vi "GEA2 Write ERD.vi"(0 "GEA2 Reference In":refnum<k24>, 1 "Retry Count":i32=5, 2 "Read Timeout (ms)":u32=500, 5 "GEA Inputs":T1 {"Destination" format="%.0x"; "Source" format="%.0x"}, 7 "Write ERD List":T2[](array[typedef]) {"ERD Number" format="%.0x"}, 11 "Error In":errorcluster, 13 "Verify ERD Response?":bool=TRUE) -> (4 "GEA2 Reference Out":refnum<k24>, 6 "Raw Data Out":string, 15 "Error Out":errorcluster)   [LabVIEW 2016, in "GEA2_Toolkit.lvlib"]
doc: "This VI writes an array of ERDs with a single command. The data type is used to convert the Data from the type specified to a hexidecimal string before sending it."
uses:
  library/GEA2_Toolkit.lvlib
  type defs/ERD Write Data In.ctl
  type defs/Data Type.ctl
  type defs/Source_Destination.ctl
  C:/TechnologyLab/NI-2010/Trunk/Utility/LabVIEW GEA2 Toolkit v1.0.0.0/Appliance.NET/GeaCommunication.dll
  Appliance.NET/GeaCommunication.dll
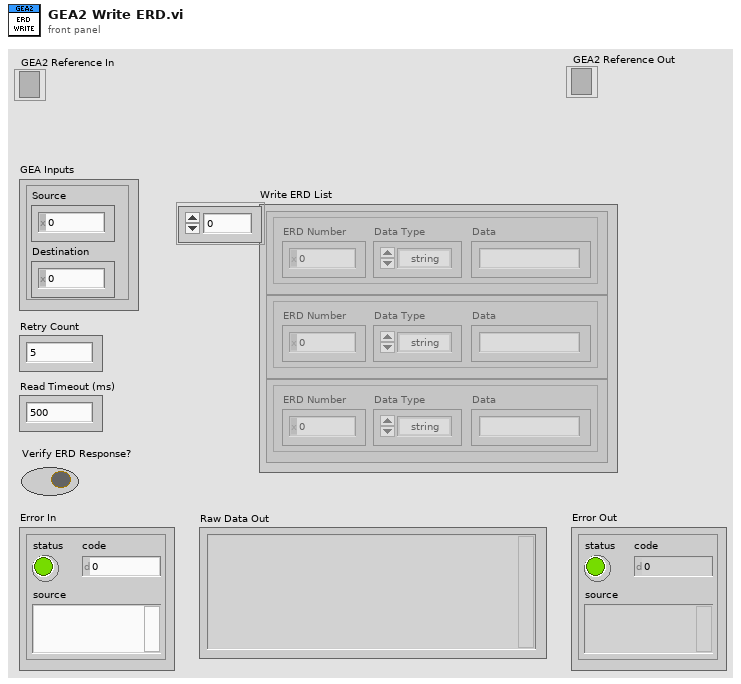
[diagram p1: front panel]
types:
  T1 = typedef "GEA2_Toolkit.lvlib/Source_Destination.ctl" = cluster{"Source":u8, "Destination":u8}
  T2 = typedef "GEA2_Toolkit.lvlib/ERD Write Data In.ctl" = cluster{"ERD Number":u16, "Data Type":T3, "Data":string}
  T3 = typedef "GEA2_Toolkit.lvlib/Data Type.ctl" = enum16{"string", "boolean", "uint8_t", "uint16_t", "uint32_t", "uint64_t"}
  T4 = typedef "GEA2_Toolkit.lvlib/Data In.ctl" = cluster{"Source":u8, "Destination":u8, "Command":u8, "Message":string}
  T5 = typedef "GEA2_Toolkit.lvlib/Data Out.ctl" = cluster{"Source":u8, "Destination":u8, "Command":u8, "Length":u8, "CRC":u16, "Message":string}
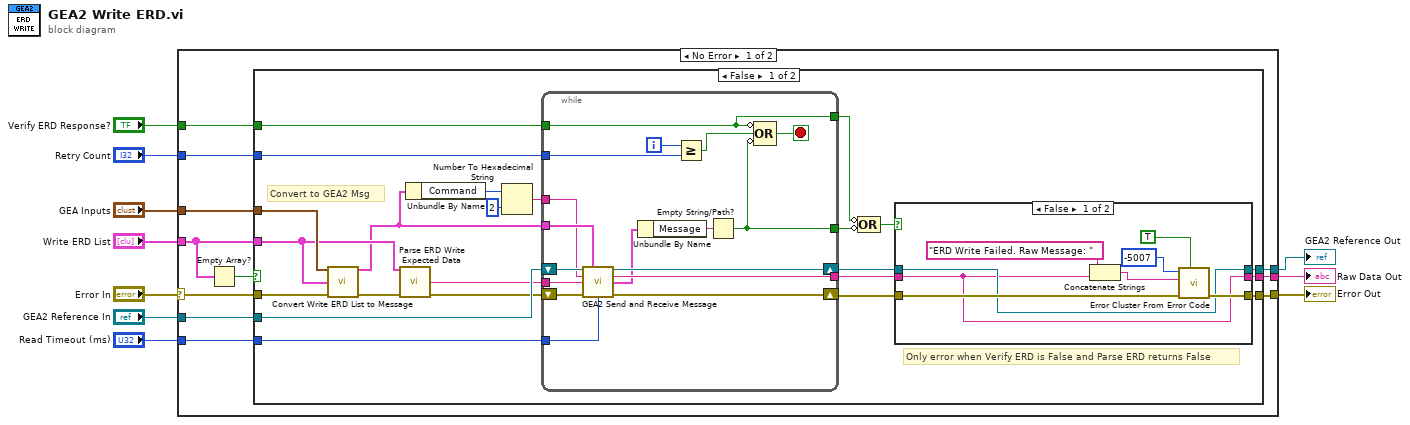
[diagram p0: block diagram]
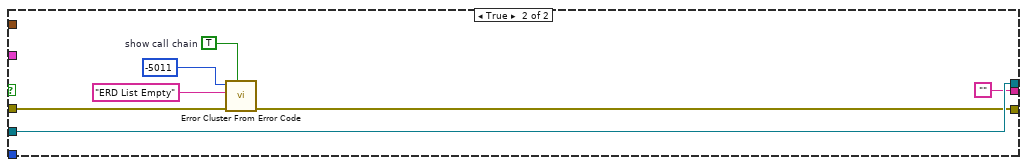
[diagram p3: hidden frame]
diagram:
  n1 = case shown="No Error" "Error In" {
    selector: "Error In" -> [w14 w80]
    tunnel: "GEA2 Reference In" -> [w13 w81]
    tunnel: "Write ERD List" -> [w12 _]
    tunnel: "Verify ERD Response?" -> [w21 _]
    tunnel: "GEA Inputs" -> [w15 _]
    tunnel: [w17 _] -> w6
    tunnel: [w18 w80] -> w5
    tunnel: "Read Timeout (ms)" -> [w20 _]
    tunnel: "Retry Count" -> [w19 _]
    tunnel: [w16 w81] -> w2
    frame No Error {
      n2 = Empty Array?(array=w12) -> (empty?=w11:bool)
      n3 = case shown="False" w11 {
        tunnel: w21 -> [w44 _]
        tunnel: w20 -> [w43 _]
        tunnel: w19 -> [w42 _]
        tunnel: [w40 w74] -> w18
        tunnel: [w39 ""] -> w17
        tunnel: [w36 w79] -> w16
        tunnel: w15 -> [w32 _]
        tunnel: w14 -> [w31 w78]
        tunnel: w13 -> [w30 w79]
        tunnel: w12 -> [w26 _]
        frame False {
          # "Only error when Verify ERD is False and Parse ERD returns False"
          # "Convert to GEA2 Msg"
          n4 = call "Convert Write ERD List to Message.vi"("GEA Inputs"=w32, "Write ERD List"=w26, "Error In"=w31) -> ("GEA Message"=w23:T4, "Error Out"=w29:errorcluster)  [unwired: 11 in]
          n5 = call "Parse ERD Write Expected Data.vi"("Write ERD List"=w26, "Error In"=w29) -> ("Expected Data"=w27:string, "Error Out"=w28:errorcluster)  [unwired: 12 in]
          n6 = Unbundle By Name(w23) -> ("Command"=w25:u8)
          n7 = Number To Hexadecimal String(1:i16 2 ("width (-)"), 2:w25) -> (0:w22:string)
          n8 = while {
            tunnel: w23 -> [w63]
            tunnel: [w72] -> w38
            tunnel: w44 -> [w64]
            tunnel: w43 -> [w70]
            tunnel: w42 -> [w68]
            tunnel: [w60] -> w34
            tunnel: [w64] -> w35
            shift-right: [w71] -> w41
            shift-left: w28 -> [w56]
            shift-right: [w65] -> w37
            shift-left: w30 -> [w59]
            tunnel: w27 -> [w58]
            tunnel: w22 -> [w57]
            i -> [w69]
            stop <- w66 stop-if-true
            n9 = call "GEA2 Send and Receive Message.vi"("GEA2 Reference In"=w59, "Input Data"=w63, "Read Timeout (ms)"=w70, "Expected Command"=w57, "Expected Data"=w58, "Error In"=w56) -> ("GEA2 Reference Out"=w65:refnum<k24>, "Raw Data Out"=w72:string, "Converted Data Out"=w62:T5, "Error Out"=w71:errorcluster)  [unwired: 4 in, 2 out]
            n10 = Unbundle By Name(w62) -> ("Message"=w61:string)
            n11 = Greater Or Equal?(x=w69, y=w68) -> (x >= y?=w67:bool)
            n12 = Empty String/Path?(string/path=w61) -> (empty?=w60:bool)
            n13 = Compound Arithmetic op=OR(invert w64, w67, invert w60) -> (w66:bool)
          }
          n14 = Compound Arithmetic op=OR(invert w35, invert w34) -> (w33:bool)
          n15 = case shown="False" w33 {
            tunnel: w41 -> [w52 w55]
            tunnel: [w51 w55] -> w40
            tunnel: [w45 w54] -> w39
            tunnel: w38 -> [w45 w54]
            tunnel: w37 -> [w48 w53]
            tunnel: [w48 w53] -> w36
            frame False {
              n16 = Concatenate Strings("ERD Write Failed. Raw Message: " ("error message (\"\")"), w45) -> (w46:string)
              n17 = call <vilib>:"Error Cluster From Error Code.vi"("show call chain? (False)"=TRUE, "error in (no error)"=w52, "error message (\"\")"=w46, "error code (0)"=-5007) -> ("error out"=w51:errorcluster)  [unwired: 5 in]
            }
            frame True {
            }
          }
        }
        frame True {
          w75 = TRUE  # show call chain
          n18 = call <vilib>:"Error Cluster From Error Code.vi"("show call chain? (False)"=w75, "error in (no error)"=w78, "error message (\"\")"="ERD List Empty" ("error message (\"\")"), "error code (0)"=-5011) -> ("error out"=w74:errorcluster)  [unwired: 5 in]
        }
      }
    }
    frame Error {
    }
  }
  "Raw Data Out" <- w6
  "Error Out" <- w5
  "GEA2 Reference Out" <- w2
